vi "Device VI 1.6.vi"() -> ()   [LabVIEW 2017]
uses:
  <vilib>/Utility/error.llb/DialogType.ctl
  <vilib>/DAQmx/read.llb/DAQmx Read (Analog 1D Wfm NChan NSamp).vi
  <vilib>/DAQmx/create/channels.llb/DAQmx Create Channel (AI-Force-Bridge-Two-Point-Linear).vi
  <vilib>/DAQmx/configure/timing.llb/DAQmx Timing (Sample Clock).vi
  <vilib>/DAQmx/configure/trigger.llb/DAQmx Start Trigger (Digital Edge).vi
  <vilib>/DAQmx/miscellaneous.llb/DAQmx Fill In Error Info.vi
  <vilib>/Waveform/WDTFileIO.llb/Export Waveforms To Spreadsheet File (1D).vi
  <resource>/objmgr/daqmx.rc
panel:
  in  "scaling information":T1={"first electrical value"=0.0, "second electrical value"=1.0, "electrical units"=15897, "first physical value"=0.0, "second physical value"=7.39, "physical units"=15876} {"physical units" items=["Newtons"=15875, "Pounds"=15876, "kgf"=15877]; "electrical units" items=["Volts/Volt"=15896, "mVolts/Volt"=15897]}
  in  "Pause":bool
  in  "Start":bool
  in  "Stop 3":bool
  in  "Spreadsheet Location":path=path "C:/Users/Julio/Desktop/Device Data/Test.xlsx" caption="Filename"
  in  "Maximum Force":dbl=25.0
  in  "Minimum Force":dbl=-25.0
  in  "Units (Force)":i32(ring)=15876 items=["Newtons"=15875, "Pounds"=15876, "kgf"=15877, "From Custom Scale"=10065]
  in  "Trigger Type":T2(tab)
  in  "Digital Start Trigger Edge":i32(ring)=10280 caption="Edge" items=["Rising"=10280, "Falling"=10171]
  in  "Digital Start Trigger Source":tag="/cDAQ1Mod3/PFI0" caption="Source"
  in  "Digital Pause Trigger Pause When":i32(ring)=10192 caption="Pause When" items=["High"=10192, "Low"=10214]
  in  "Digital Pause Trigger Source":tag="/Dev1/PFI0" caption="Source"
  in  "Bridge Information":T3={"Bridge Configuration"=10182, "Excitation Source"=10200, "Excitation Value"=10.0, "Nominal Resistance"=350.0} {"Excitation Source" items=["Internal"=10200, "External"=10167, "None"=10230]; "Bridge Configuration" items=["Full Bridge"=10182, "Half Bridge"=10187, "Quarter Bridge"=10270, "No Bridge"=10228]}
  in  "Physical Channel":tag="cDAQ1Mod1/ai0:1"
  in  "Sample Rate":dbl=1000.0
  in  "Samples per Loop":i32=500
  out "Waveform Chart":waveform(dbl)[](graph)=[{"t0"=timestamp(3613388787.7661867 s since 1904-01-01), "dt"=0.00062, "Y"=array[500 elements], "attributes"=variant("NI_ChannelName"=variant(string "cDAQ1Mod1/ai0"), "NI_UnitDescription"=variant(string "Pounds"))}, {"t0"=timestamp(3613388787.7661867 s since 1904-01-01), "dt"=0.00062, "Y"=array[500 elements], "attributes"=variant("NI_ChannelName"=variant(string "cDAQ1Mod1/ai1"), "NI_UnitDescription"=variant(string "Pounds"))}]
  # "Settings"
  # "Data"
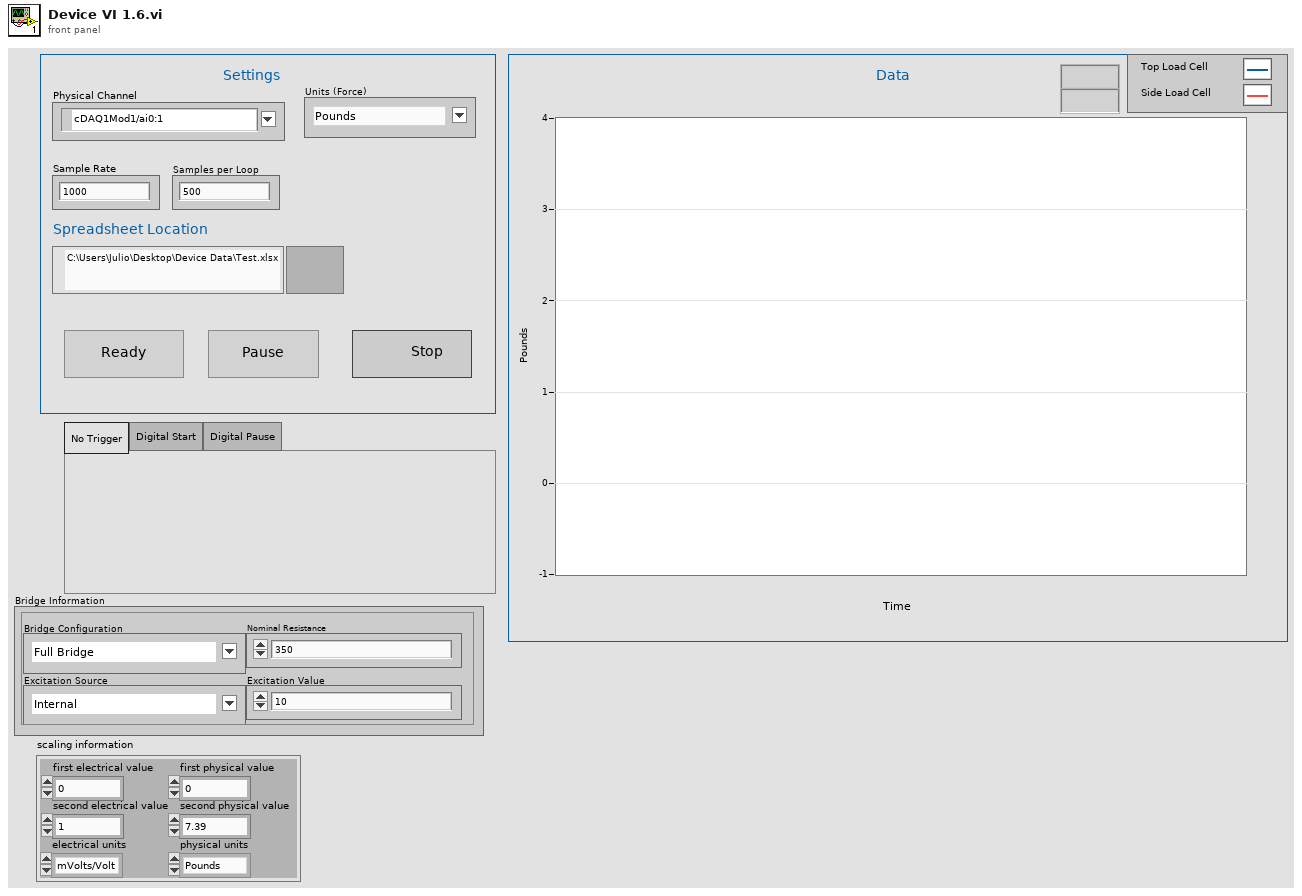
[diagram p1: front panel]
types:
  T1 = cluster{"first electrical value":dbl, "second electrical value":dbl, "electrical units":i32, "first physical value":dbl, "second physical value":dbl, "physical units":i32}
  T2 = enum32{"No Trigger", "Digital Start", "Digital Pause"}
  T3 = cluster{"Bridge Configuration":i32, "Excitation Source":i32, "Excitation Value":dbl, "Nominal Resistance":dbl}
  T4 = typedef "DialogType.ctl" = u16
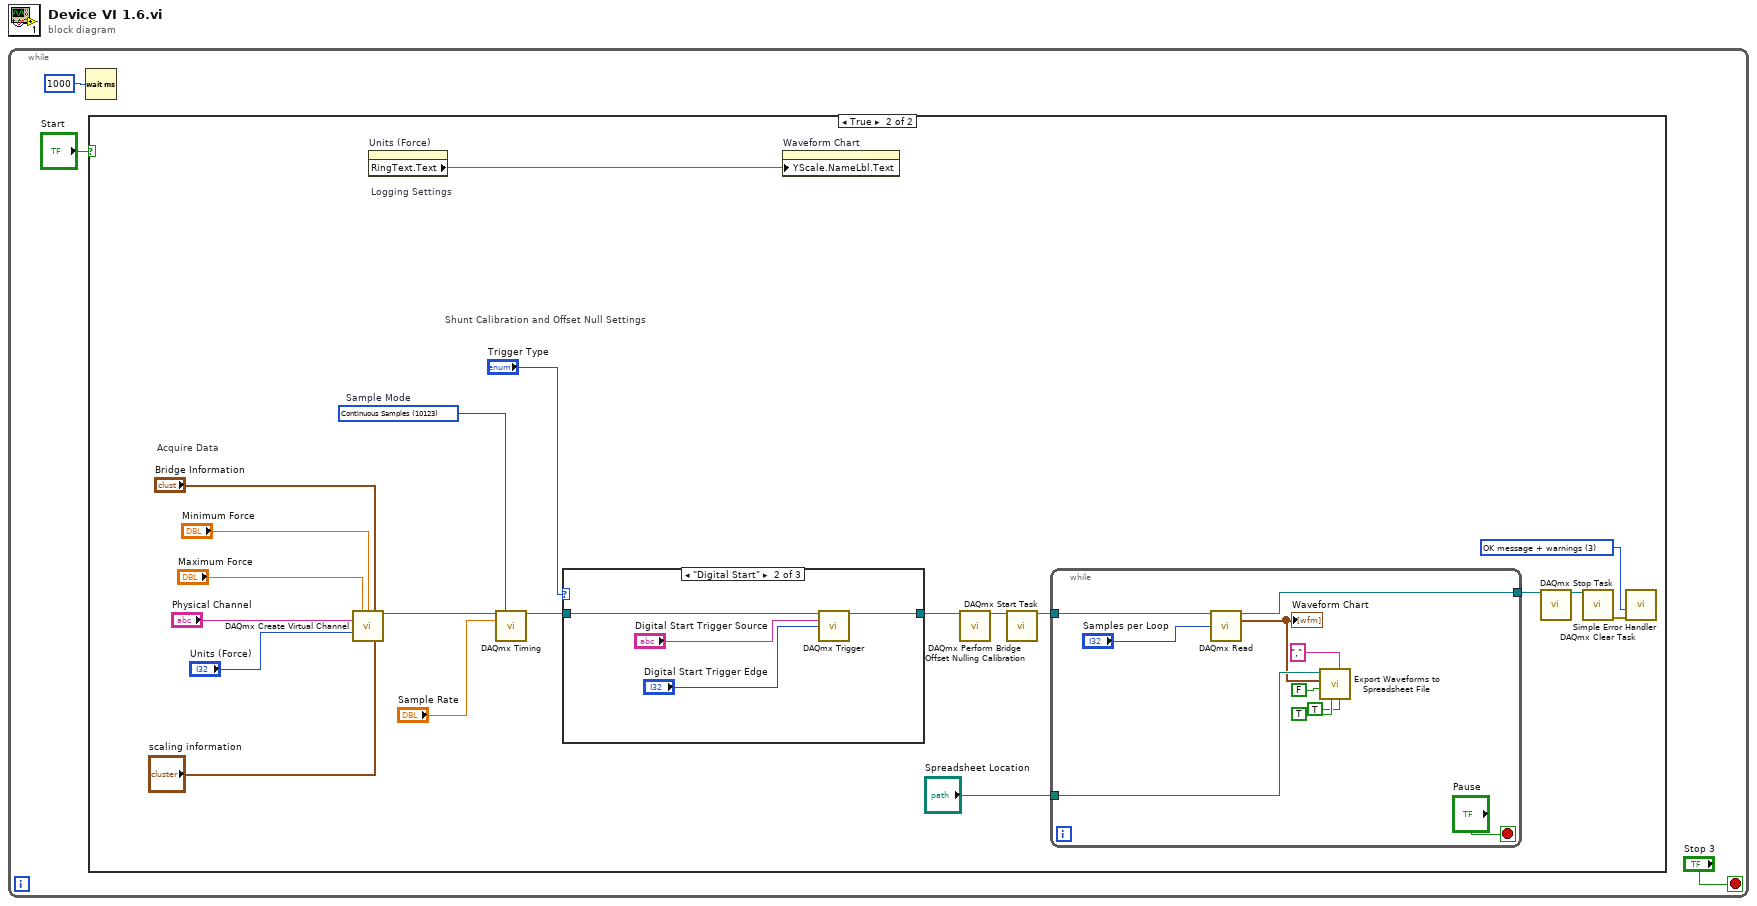
[diagram p0: block diagram]
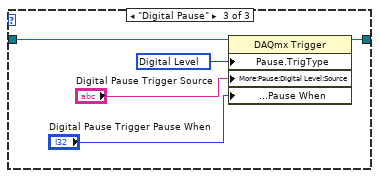
[diagram p4: hidden frame]
diagram:
  n1 = while {
    stop <- "Stop 3" stop-if-true
    n2 = Wait (ms)(milliseconds to wait=u32 1000) -> ()  [unwired: 1 out]
    n3 = case shown="True" "Start" {
      frame False {
      }
      frame True {
        w15 = T4 3 items=["no dialog", "OK message", "continue or stop message", "OK message + warnings", "continue/stop + warnings"] ("type of dialog (OK msg:1)")
        w23 = 10123 items=["Finite Samples"=10178, "Continuous Samples"=10123, "Hardware Timed Single Point"=12522]  # Sample Mode
        # "Logging Settings"
        # "Acquire Data"
        # "Shunt Calibration and Offset Null Settings"
        n4 = call-poly <vilib>:"DAQmx Create Virtual Channel.vi"("maximum value"="Maximum Force", "minimum value"="Minimum Force", "bridge information"="Bridge Information", "physical channels"="Physical Channel", "units"="Units (Force)", "scaling information"="scaling information") -> ("task out"=w22:refnum<k21>)  [unwired: 8 in, 1 out]
        n5 = property on="Units (Force)" class="Ring (strict)"() -> ("RingText.Text"=w8:string)  [unwired: 2 in, 2 out]
        n6 = call-poly <vilib>:"DAQmx Timing.vi"("task/channels in"=w22, "sample mode"=w23, "rate"="Sample Rate") -> ("task out"=w9:refnum<k21>)  [unwired: 11 in, 1 out]
        n7 = case shown="\"Digital Start\"" "Trigger Type" {
          tunnel: w9 -> [w24 w28 w33]
          tunnel: [w24 w27 w32] -> w13
          frame "No Trigger", Default {
          }
          frame "Digital Start" {
            n8 = call-poly <vilib>:"DAQmx Trigger.vi"("task/channels in"=w28, "source"="Digital Start Trigger Source", "edge"="Digital Start Trigger Edge") -> ("task out"=w27:refnum<k21>)  [unwired: 11 in, 1 out]
          }
          frame "Digital Pause" {
            w31 = 10152 items=["Analog Level"=10101, "Analog Window"=10103, "Digital Level"=10152, "Digital Pattern"=10398, "None"=10230] ("Pause.TrigType")
            n9 = property class="DAQmx Trigger"(reference=w33, "Pause.TrigType"=w31, "More:Pause:Digital Level:Source"="Digital Pause Trigger Source", "More:Pause:Digital Level:Pause When"="Digital Pause Trigger Pause When") -> (reference out=w32:refnum<k21>)  [unwired: 1 in, 1 out]
          }
        }
        n10 = property on="Waveform Chart" class="WFChart (strict)"("YScale.NameLbl.Text"=w8) -> ()  [unwired: 2 in, 2 out]
        n11 = call <vilib>:"DAQmx Perform Bridge Offset Nulling Calibration.vi"("task/channels in"=w13) -> ("task out"=w7:refnum<k21>)  [unwired: 13 in, 1 out]
        n12 = call <vilib>:"DAQmx Start Task.vi"("task/channels in"=w7) -> ("task out"=w21:refnum<k21>)  [unwired: 13 in, 1 out]
        n13 = while {
          tunnel: w21 -> [w43]
          tunnel: "Spreadsheet Location" -> [w40]
          tunnel: [w35] -> w4
          stop <- "Pause" stop-if-true
          n14 = call-poly <vilib>:"DAQmx Read.vi"("task/channels in"=w43, "number of samples per channel"="Samples per Loop") -> ("task out"=w35:refnum<k21>, "data"=w39:waveform(dbl)[])  [unwired: 11 in, 1 out]
          "Waveform Chart" <- w39
          n15 = call-poly <vilib>:"Export Waveforms to Spreadsheet File.vi"("header? (write header:T)"=TRUE, "delimiter (Tab)"=",", "append to file? (new file:F)"=TRUE, "multiple time columns? (single:F)"=FALSE, "waveforms"=w39, "file path (dialog if empty)"=w40) -> ()  [unwired: 4 in, 2 out]
        }
        n16 = call <vilib>:"DAQmx Stop Task.vi"("task/channels in"=w4) -> ("task out"=w16:refnum<k21>)  [unwired: 13 in, 1 out]
        n17 = call <vilib>:"DAQmx Clear Task.vi"("task in"=w16) -> ("error out"=w20:errorcluster)  [unwired: 14 in]
        n18 = call <vilib>:"Simple Error Handler.vi"("type of dialog (OK msg:1)"=w15, "error in (no error)"=w20) -> ()  [unwired: 3 in, 5 out]
      }
    }
  }
